vi "FL Set Membership Function (MF array).vi"(0 "membership functions in":T1[](array[typedef]) {"shape" items=["Triangle", "Trapezoid", "Singleton", "Sigmoid", "Gaussian", "User-Defined"]}, 3 "membership function index":i32, 5 "name":string, 7 "shape":T2 items=["Triangle", "Trapezoid", "Singleton", "Sigmoid", "Gaussian", "User-Defined"], 9 "points":dbl[](array[numeric]), 11 "error in (no error)":errorcluster, 12 "color":u32(colorbox)=16777215, 13 "user-defined membership function shapes":cluster{"Y":dbl[], "X":dbl[]}[](array[cluster]), 14 "user-defined \nshape index":i32) -> (4 "membership functions out":T1[](array[typedef]) {"shape" items=["Triangle", "Trapezoid", "Singleton", "Sigmoid", "Gaussian", "User-Defined"]}, 15 "error out":errorcluster)   [LabVIEW 2017, in "NI_Fuzzy_Logic_API.lvlib"]
doc: "Modifies the shape, color, or points of a membership function for a linguistic variable. You can modify a membership function from a fuzzy system or from an array of membership functions. The data type you wire to the <B>fuzzy system in</B> input determines the polymorphic instance to use."
uses:
  <vilib>/addons/Fuzzy Logic/NI_Fuzzy_Logic_API.lvlib
  <vilib>/addons/Fuzzy Logic/TypeDefs/FL Membership Function Shape.ctl
  <vilib>/addons/Fuzzy Logic/TypeDefs/FL Membership Function.ctl
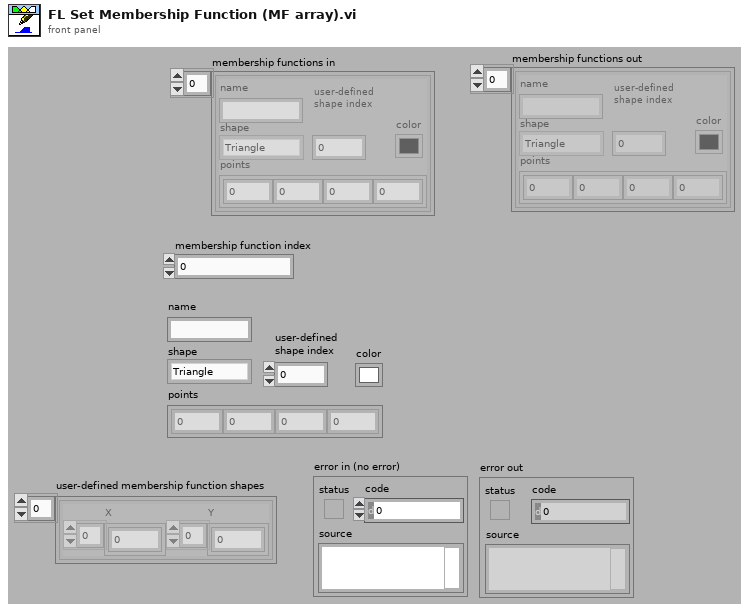
[diagram p1: front panel]
types:
  T1 = typedef "NI_Fuzzy_Logic_API.lvlib/FL Membership Function.ctl" = cluster{"name":string, "shape":T2, "points":dbl[], "color":u32, "user-defined shape index":i32}
  T2 = typedef "NI_Fuzzy_Logic_API.lvlib/FL Membership Function Shape.ctl" = u16
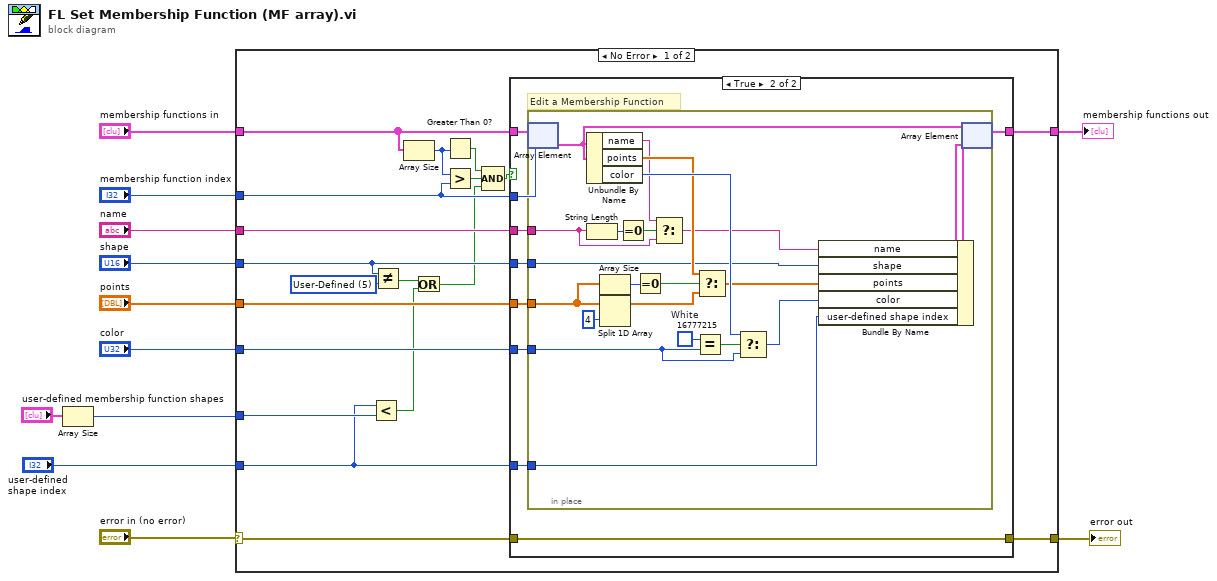
[diagram p0: block diagram]
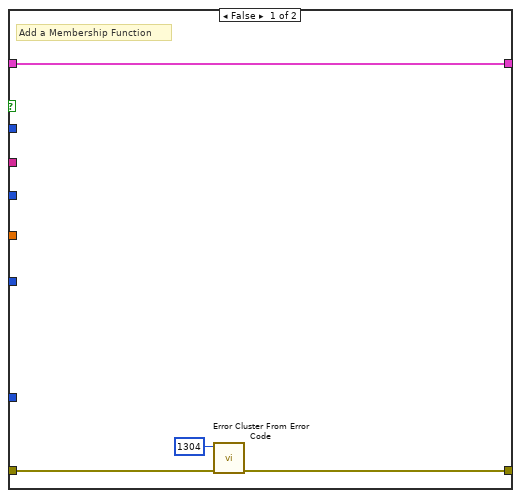
[diagram p2: hidden frame]
diagram:
  n1 = Array Size(array="user-defined membership function shapes") -> (size(s)=w2:i32)
  n2 = case shown="No Error" "error in (no error)" {
    selector: "error in (no error)" -> [w21 w67]
    tunnel: "membership function index" -> [w31 _]
    tunnel: "name" -> [w30 _]
    tunnel: "shape" -> [w18 _]
    tunnel: "color" -> [w29 _]
    tunnel: "points" -> [w28 _]
    tunnel: [w20 w67] -> w6
    tunnel: [w23 w66] -> w5
    tunnel: "membership functions in" -> [w22 w66]
    tunnel: w2 -> [w15 _]
    tunnel: "user-defined \nshape index" -> [w14 _]
    frame No Error {
      w19 = T2 5 items=["Triangle", "Trapezoid", "Singleton", "Sigmoid", "Gaussian", "User-Defined"] ("y")
      n3 = Less?(x=w14, y=w15) -> (x < y?=w13:bool)
      n4 = Not Equal?(x=w18, y=w19) -> (x != y?=w17:bool)
      n5 = Array Size(array=w22) -> (size(s)=w26:i32)
      n6 = Or(x=w17, y=w13) -> (x .or. y?=w16:bool)
      n7 = Greater Than 0?(x=w26) -> (x > 0?=w25:bool)
      n8 = Greater?(x=w26, y=w31) -> (0:w27:bool)
      n9 = Compound Arithmetic op=AND(w25, w27, w16) -> (w24:bool)
      n10 = case shown="True" w24 {
        tunnel: w31 -> [_ w42]
        tunnel: [w35 w43] -> w23
        tunnel: w22 -> [w35 w44]
        tunnel: w30 -> [_ w41]
        tunnel: w29 -> [_ w39]
        tunnel: w28 -> [_ w40]
        tunnel: w18 -> [_ w38]
        tunnel: w21 -> [w34 w37]
        tunnel: [w33 w37] -> w20
        tunnel: w14 -> [_ w36]
        frame False {
          # "Add a Membership Function"
          n11 = call <vilib>:"Error Cluster From Error Code.vi"("error in (no error)"=w34, "error code (0)"=1304) -> ("error out"=w33:errorcluster)  [unwired: 1 in, 6 out]
        }
        frame True {
          # "Edit a Membership Function"
          n12 = in-place {
            in-place-border: w40 -> [w53]
            in-place-border: w41 -> [w55]
            in-place-border: w39 -> [w54]
            in-place-border: w38 -> [w48]
            in-place-border: w36 -> [w45]
            w61 = u32 16777215  # White
            n13 = in-place-array #1(w44, w42) -> (w46:T1)
            n14 = Unbundle By Name(w46) -> ("name"=w59:string, "points"=w63:dbl[], "color"=w64:u32)
            n15 = String Length(string=w55) -> (length=w58:i32)
            n16 = Array Size(array=w53) -> (size(s)=w65:i32)
            n17 = Split 1D Array(array=w53, index=4) -> (first subarray=w51:dbl[])  [unwired: 1 out]
            n18 = Equal To 0?(x=w58) -> (x = 0?=w57:bool)
            n19 = Equal To 0?(x=w65) -> (x = 0?=w60:bool)
            n20 = Select(t=w59, s=w57, f=w55) -> (s? t:f=w47:string)
            n21 = Equal?(x=w61, y=w54) -> (x = y?=w62:bool)
            n22 = Select(t=w63, s=w60, f=w51) -> (s? t:f=w49:dbl[])
            n23 = Select(t=w64, s=w62, f=w54) -> (s? t:f=w50:u32)
            n24 = Bundle By Name(cluster=w46, "name"=w47, "shape"=w48, "points"=w49, "color"=w50, "user-defined shape index"=w45) -> (w56:T1)
            n25 = in-place-array #1(w56) -> (w43:T1[])  [unwired: 1 out]
          }
        }
      }
    }
    frame Error {
    }
  }
  "error out" <- w6
  "membership functions out" <- w5
